vi "Pause VIs in Response to User Event.vi"(8 "error in":errorcluster, 10 "VI":string, 11 "Configuration In":T1) -> (0 "error out":errorcluster)   [LabVIEW 2013, in "LVTM.lvlib"]
uses:
  LVTM.lvlib
  Controls_LVTM/LVTM_Config_Info.ctl
  Controls_LVTM/View.ctl
  Controls_LVTM/SharedDataDVR.ctl
  Pause Action.ctl
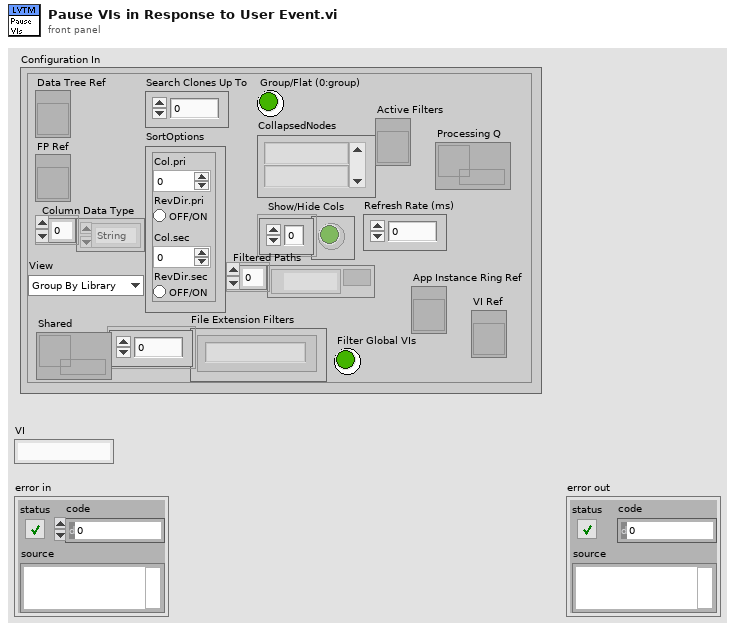
[diagram p1: front panel]
types:
  T1 = typedef "LVTM.lvlib/LVTM_Config_Info.ctl" = cluster{"Data Tree Ref":refnum<vi>, "FP Ref":refnum<vi>, "Column Data Type":enum16{"String", "Numeric"}[], "Search Clones Up To":i32, "SortOptions":cluster{"Col.pri":i32, "RevDir.pri":bool, "Col.sec":i32, "RevDir.sec":bool}, "Group/Flat (0:group)":bool, "CollapsedNodes":string[], "Show/Hide Cols":bool[], "Filtered Paths":path[], "View":T2, "File Extension Filters":string[], "Filter Global VIs":bool, "Shared":refnum<data-value>, "Active Filters":refnum<vi>, "Refresh Rate (ms)":i32, "App Instance Ring Ref":refnum<vi>, "Processing Q":refnum<queue>, "VI Ref":refnum<vi>}
  T2 = typedef "LVTM.lvlib/View.ctl" = enum16{"Group By Library", "Group By Folder", "Flat List"}
  T3 = typedef "LVTM.lvlib/Pause Action.ctl" = enum16{"Pause", "Resume", "Toggle Pause"}
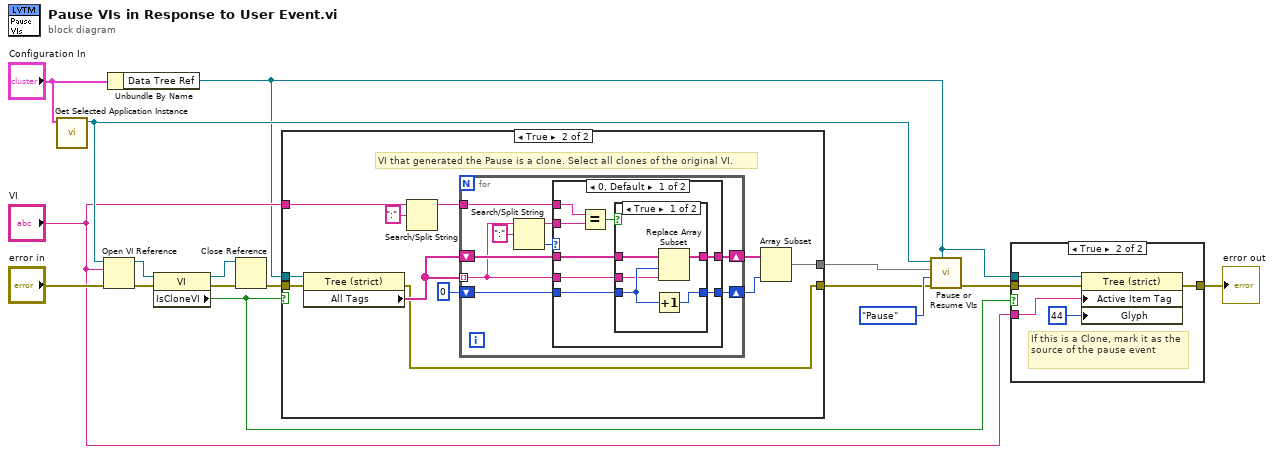
[diagram p0: block diagram]
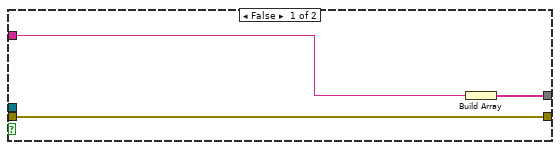
[diagram p2: hidden frame]
diagram:
  n1 = call "Get Selected Application Instance.vi"("Configuration"="Configuration In") -> ("Application out"=w14:refnum<vi>)  [unwired: 10 in]
  n2 = Open VI Reference(application reference (local)=w14, vi path="VI", error in (no error)="error in") -> (vi reference=w3:refnum<vi>, error out=w4:errorcluster)  [unwired: 3 out]
  n3 = Unbundle By Name("Configuration In") -> ("Data Tree Ref"=w2:refnum<vi>)
  n4 = property class="VI"(reference=w3, error in=w4) -> (reference out=w6:refnum<vi>, error out=w5:errorcluster, "IsCloneVI"=w8:bool)
  n5 = Close Reference(reference=w6, error in (no error)=w5) -> (error out=w7:errorcluster)
  n6 = case shown="True" w8 {
    tunnel: "VI" -> [w18 w29]
    tunnel: [w19 w23] -> w12
    tunnel: w7 -> [w17 w21]
    tunnel: w2 -> [_ w22]
    tunnel: [w17 w20] -> w1
    frame False {
      n7 = Build Array(w18) -> (w19:string[])
    }
    frame True {
      # "VI that generated the Pause is a clone. Select all clones of the original VI."
      n8 = property on="Property Node" class="Tree (strict)"(reference=w22, error in=w21) -> (error out=w20:errorcluster, "All Tags"=w24:string[])  [unwired: 1 out]
      n9 = Search/Split String(string=w29, search string/char (-)=":") -> (substring before match=w25:string)  [unwired: 1 in, 2 out]
      n10 = for {
        shift-right: [w38] -> w27
        shift-left: w24 -> [w39]
        tunnel: w24 -> [w34] mode=indexing
        shift-right: [w37] -> w26
        shift-left: 0 -> [w36]
        tunnel: w25 -> [w31]
        n11 = Search/Split String(string=w34, search string/char (-)=":") -> (substring before match=w32:string, offset of match=w33:i32)  [unwired: 1 in, 1 out]
        n12 = case shown="0, Default" w33 {
          tunnel: w39 -> [w47 w56]
          tunnel: [w46 w56] -> w38
          tunnel: [w45 w55] -> w37
          tunnel: w36 -> [w44 w55]
          tunnel: w34 -> [w43 _]
          tunnel: w32 -> [w42 _]
          tunnel: w31 -> [w41 _]
          frame 0, Default {
            n13 = Equal?(x=w41, y=w42) -> (x = y?=w40:bool)
            n14 = case shown="True" w40 {
              tunnel: w47 -> [w52 w54]
              tunnel: [w49 w54] -> w46
              tunnel: [w50 w53] -> w45
              tunnel: w44 -> [w51 w53]
              tunnel: w43 -> [w48 _]
              frame True {
                n15 = Increment(x=w51) -> (x+1=w50:i32)
                n16 = Replace Array Subset(array=w52, new element=w48, index=w51) -> (w49:string[])
              }
              frame False {
              }
            }
          }
          frame -1 {
          }
        }
      }
      n17 = Array Subset(array=w27, length=w26) -> (w23:string[])  [unwired: 1 in]
    }
  }
  n18 = call "Pause or Resume VIs.vi"("Tree"=w2, "error in"=w1, "Action"=Pause_Action."Pause", "VIs"=w12, "Application in"=w14) -> ("error out"=w13:errorcluster)  [unwired: 6 in]
  n19 = case shown="True" w8 {
    tunnel: w13 -> [w57 w61]
    tunnel: "VI" -> [_ w59]
    tunnel: [w57 w60] -> w11
    tunnel: w2 -> [_ w58]
    frame False {
    }
    frame True {
      # "If this is a Clone, mark it as the source of the pause event"
      n20 = property on="Property Node" class="Tree (strict)"(reference=w58, error in=w61, "Active Item Tag"=w59, "Glyph"=44 ("Active Item:Symbol Index")) -> (error out=w60:errorcluster)  [unwired: 1 out]
    }
  }
  "error out" <- w11
